vi "main.vi"() -> ()   [LabVIEW 2015]
panel:
  in  "stop":bool
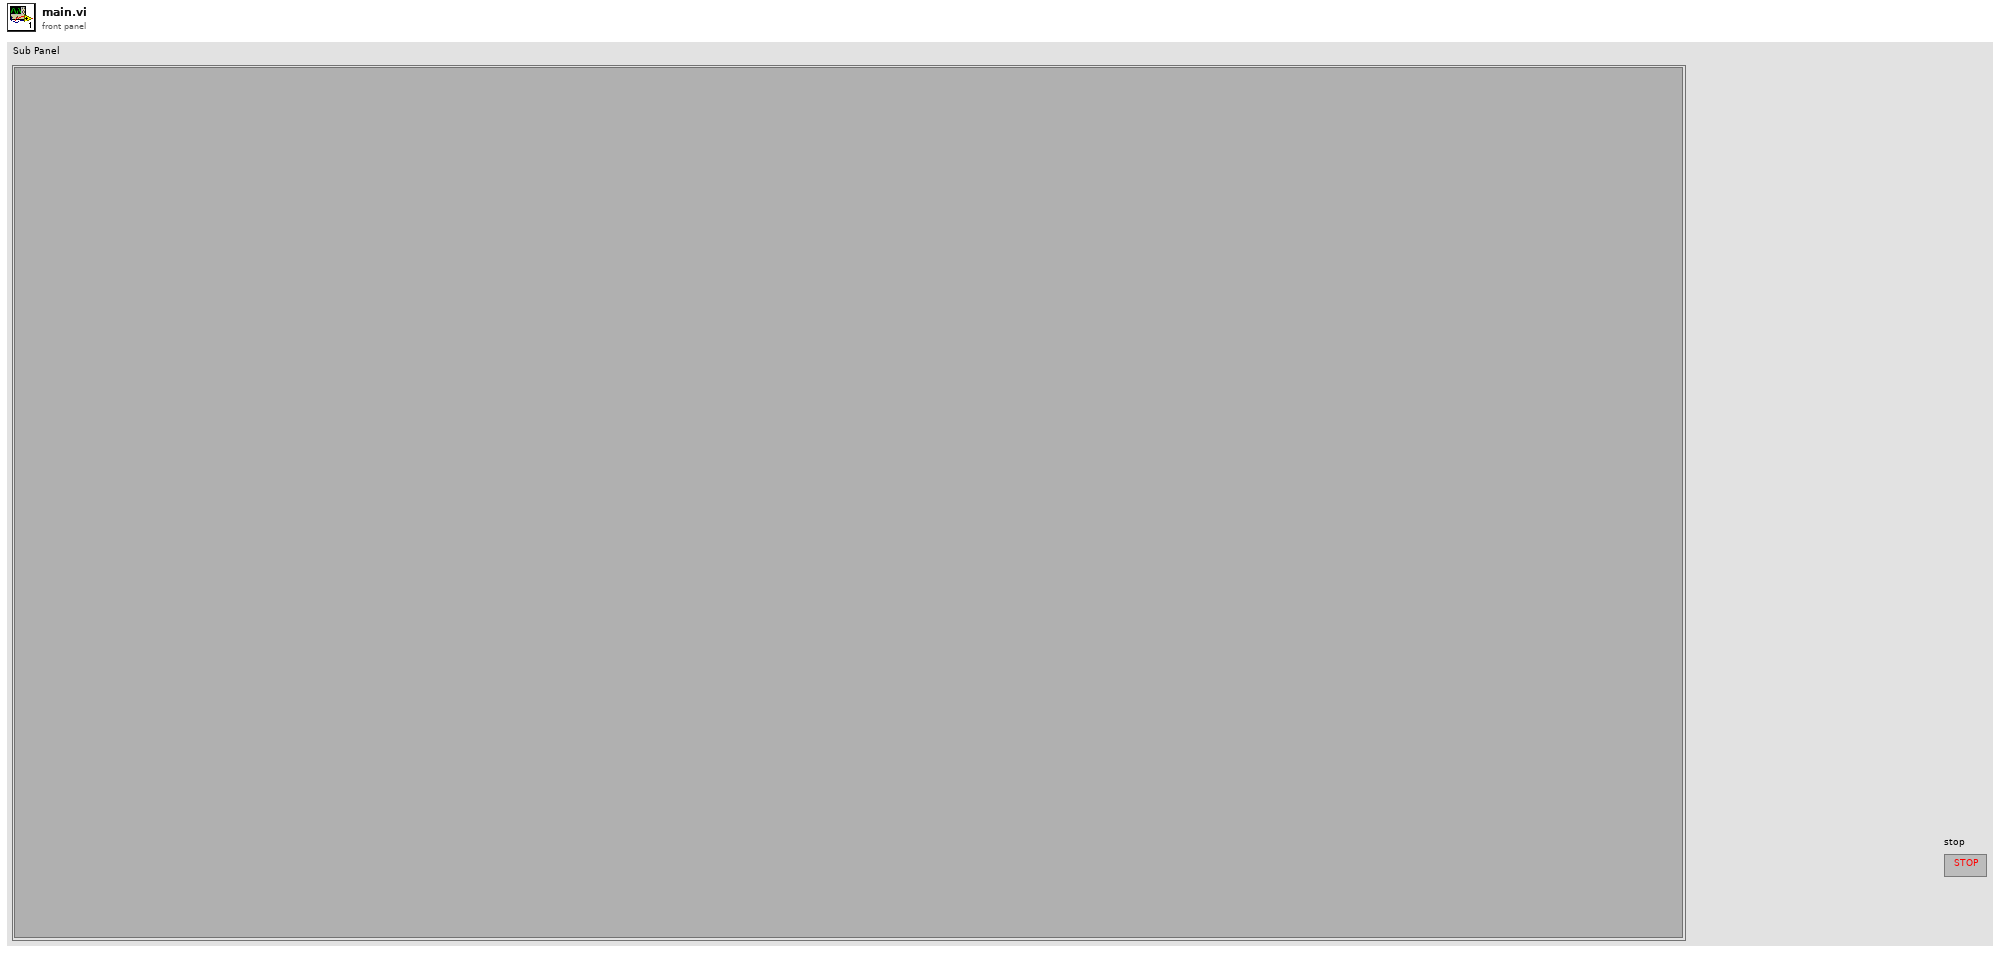
[diagram p1: front panel]
types:
  T1 = enum32{"Bad", "Idle", "Run top level", "Running"}
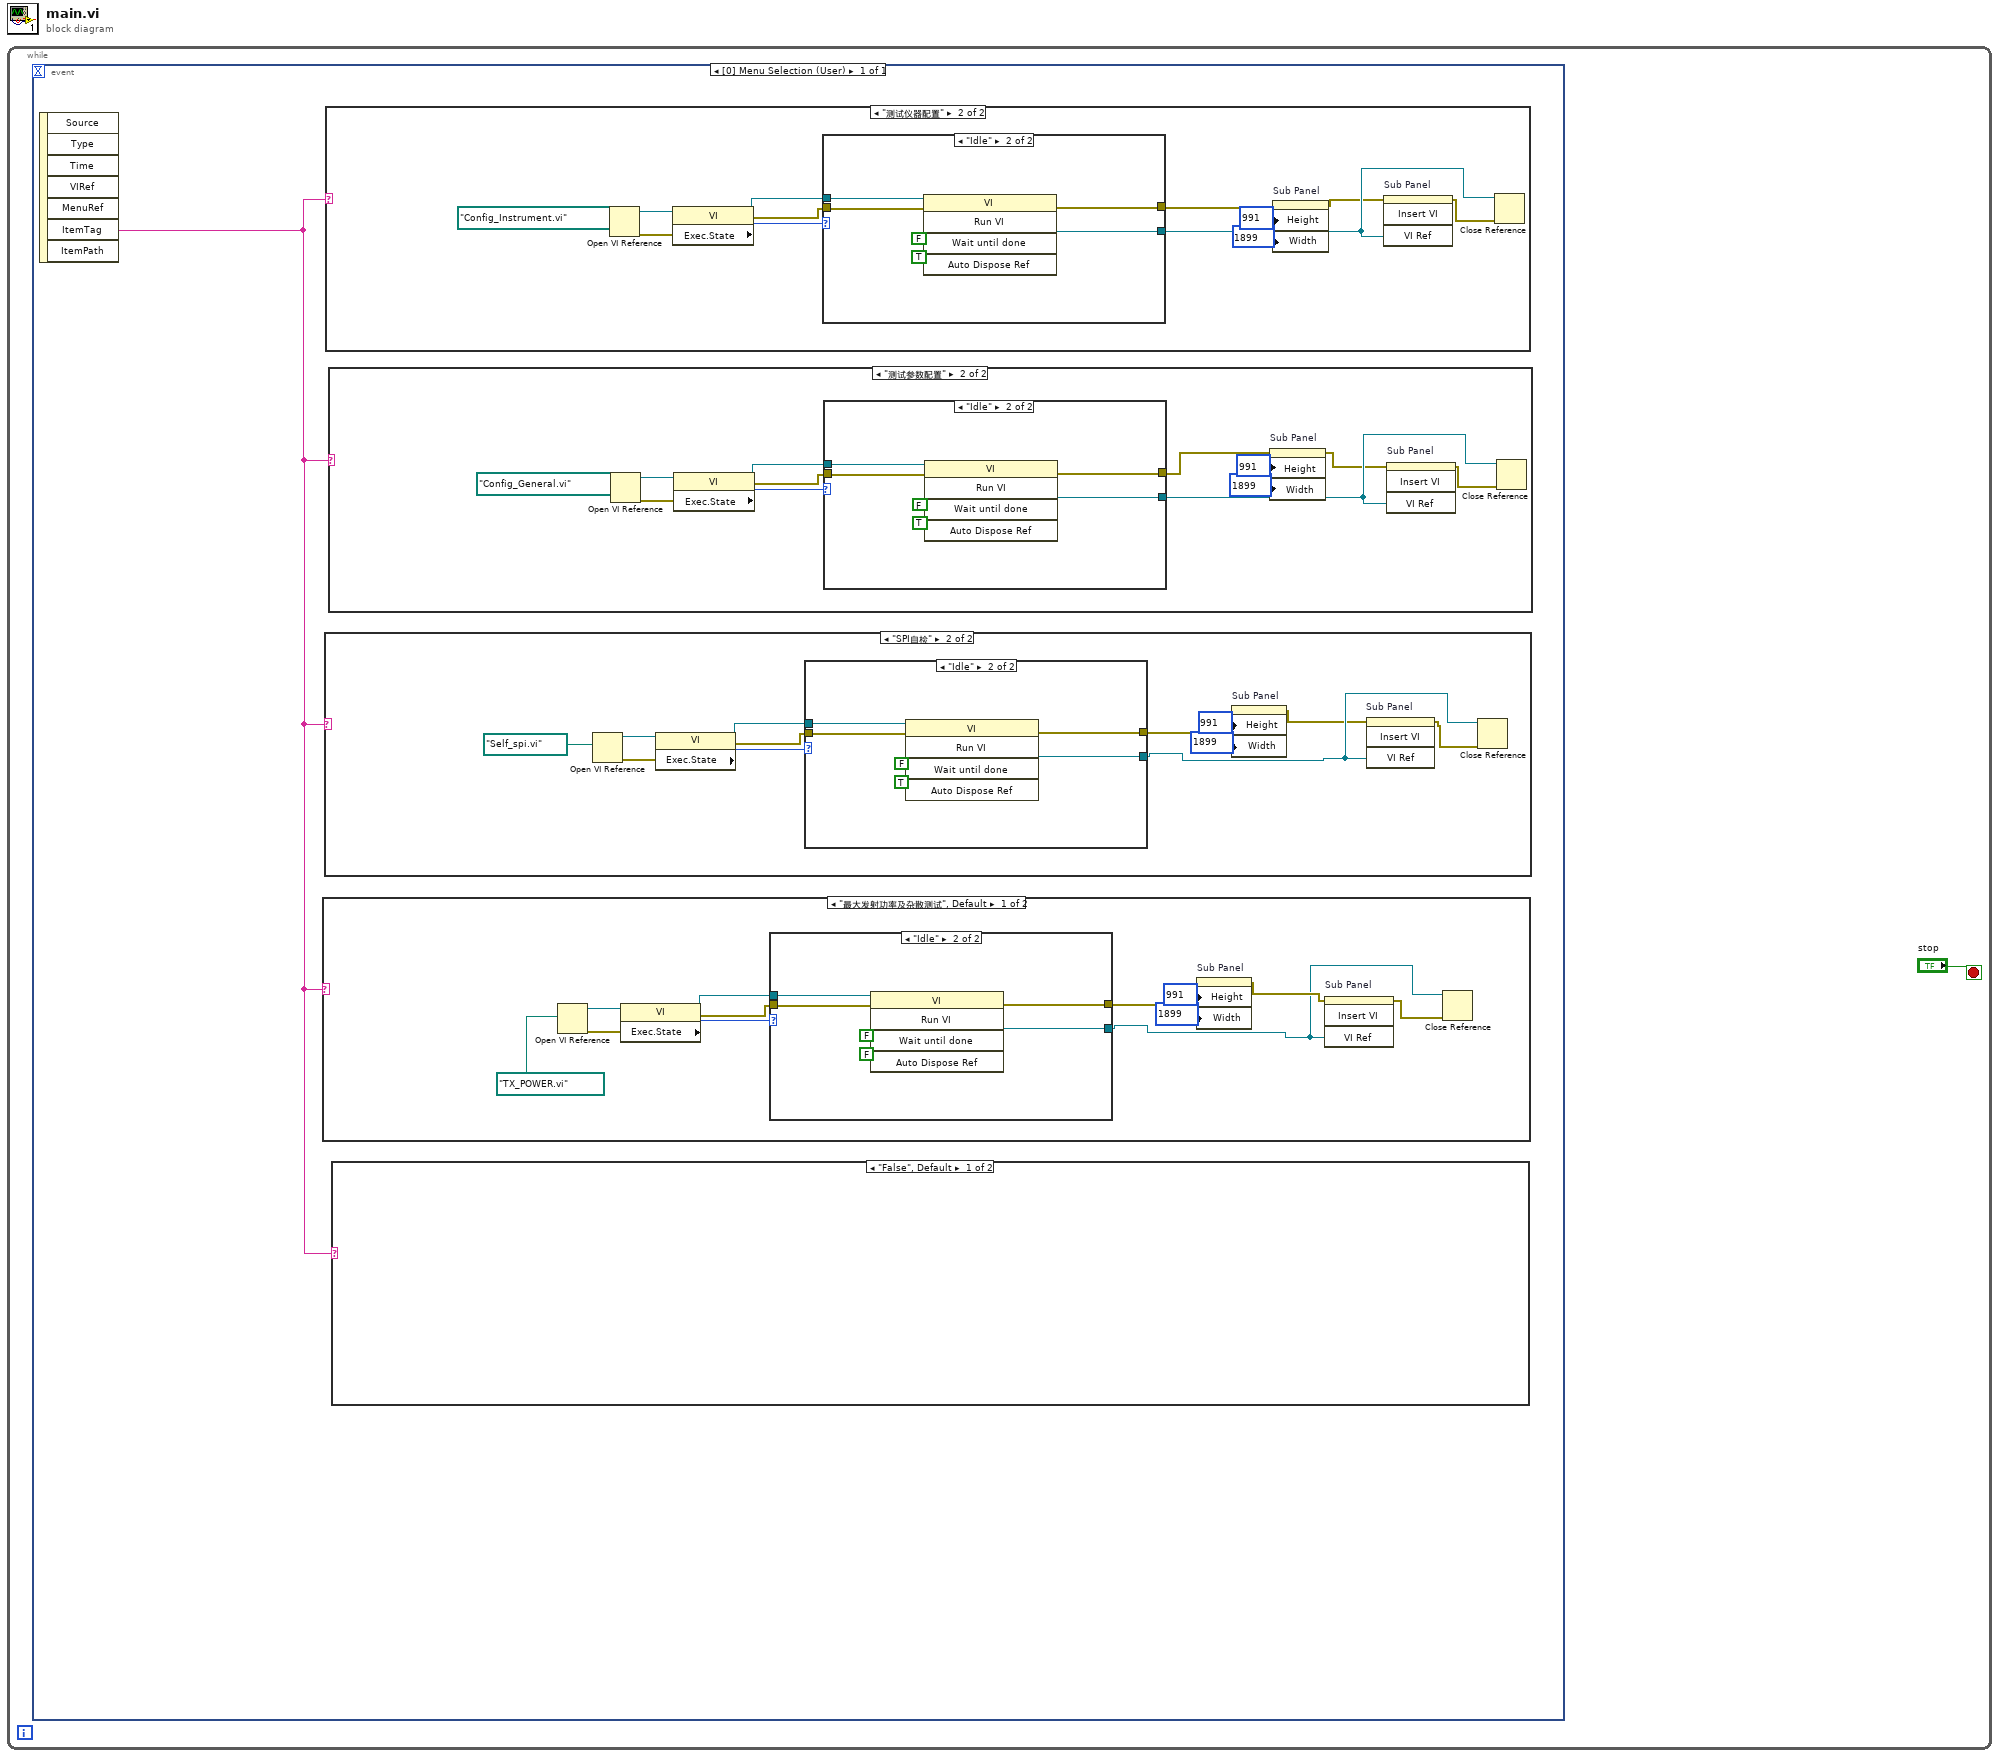
[diagram p0: block diagram]
diagram:
  n1 = while {
    stop <- "stop" stop-if-true
    n2 = event shown="[0] Menu Selection (User)" {
      selector: _ -> [_]
      dyn-events: _ -> [_]
      timeout: _ -> [_]
      event Menu Selection (User) {
        n3 = event-data() -> ("ItemTag"=w2:string)  [unwired: 1 in, 6 out]
        n4 = case shown="\"最大发射功率及杂散测试\", Default" w2 {
          frame "最大发射功率及杂散测试", Default {
            n5 = Open VI Reference(vi path=path "TX_POWER.vi") -> (vi reference=w6:refnum<vi>, error out=w8:errorcluster)  [unwired: 5 in]
            n6 = property class="VI"(reference=w6, error in=w8) -> (reference out=w9:refnum<vi>, error out=w10:errorcluster, "Exec.State"=w7:T1)
            n7 = case shown="\"Idle\"" w7 {
              tunnel: w9 -> [_ w20]
              tunnel: w10 -> [_ w19]
              tunnel: [_ w18] -> w12
              tunnel: [_ w17] -> w3
              frame "Bad", Default {
              }
              frame "Idle" {
                n8 = invoke class="VI" method="Run VI"(reference=w20, error in=w19, "Wait until done"=FALSE ("Wait Until Done"), "Auto Dispose Ref"=FALSE ("Auto Dispose Reference")) -> (reference out=w17:refnum<vi>, error out=w18:errorcluster)  [unwired: 1 in, 3 out]
              }
            }
            n9 = property on="Sub Panel" class="SubPnl"(error in=w12, "Height"=u32 991 ("Container Bounds:Height"), "Width"=u32 1899 ("Container Bounds:Width")) -> (error out=w5:errorcluster)  [unwired: 1 in, 1 out]
            n10 = invoke on="Sub Panel" class="SubPnl" method="Insert VI"(error in=w5, "VI Ref"=w3) -> (error out=w4:errorcluster)  [unwired: 2 in, 3 out]
            n11 = Close Reference(reference=w3, error in (no error)=w4) -> ()  [unwired: 1 out]
          }
          frame "2" {
          }
        }
        n12 = case shown="\"SPI自检\"" w2 {
          frame "False", Default {
          }
          frame "SPI自检" {
            n13 = Open VI Reference(vi path=path "Self_spi.vi") -> (vi reference=w32:refnum<vi>, error out=w30:errorcluster)  [unwired: 5 in]
            n14 = property class="VI"(reference=w32, error in=w30) -> (reference out=w29:refnum<vi>, error out=w28:errorcluster, "Exec.State"=w31:T1)
            n15 = case shown="\"Idle\"" w31 {
              tunnel: w29 -> [_ w38]
              tunnel: w28 -> [_ w37]
              tunnel: [_ w36] -> w24
              tunnel: [_ w35] -> w25
              frame "Bad", Default {
              }
              frame "Idle" {
                n16 = invoke class="VI" method="Run VI"(reference=w38, error in=w37, "Wait until done"=FALSE ("Wait Until Done"), "Auto Dispose Ref"=TRUE ("Auto Dispose Reference")) -> (reference out=w35:refnum<vi>, error out=w36:errorcluster)  [unwired: 1 in, 3 out]
              }
            }
            n17 = property on="Sub Panel" class="SubPnl"(error in=w24, "Height"=u32 991 ("Container Bounds:Height"), "Width"=u32 1899 ("Container Bounds:Width")) -> (error out=w23:errorcluster)  [unwired: 1 in, 1 out]
            n18 = invoke on="Sub Panel" class="SubPnl" method="Insert VI"(error in=w23, "VI Ref"=w25) -> (error out=w26:errorcluster)  [unwired: 2 in, 3 out]
            n19 = Close Reference(reference=w25, error in (no error)=w26) -> ()  [unwired: 1 out]
          }
        }
        n20 = case shown="\"测试仪器配置\"" w2 {
          frame "False", Default {
          }
          frame "测试仪器配置" {
            n21 = Open VI Reference(vi path=path "Config_Instrument.vi") -> (vi reference=w43:refnum<vi>, error out=w45:errorcluster)  [unwired: 5 in]
            n22 = property class="VI"(reference=w43, error in=w45) -> (reference out=w46:refnum<vi>, error out=w47:errorcluster, "Exec.State"=w44:T1)
            n23 = case shown="\"Idle\"" w44 {
              tunnel: w46 -> [_ w56]
              tunnel: w47 -> [_ w55]
              tunnel: [_ w54] -> w42
              tunnel: [_ w53] -> w48
              frame "Bad", Default {
              }
              frame "Idle" {
                n24 = invoke class="VI" method="Run VI"(reference=w56, error in=w55, "Wait until done"=FALSE ("Wait Until Done"), "Auto Dispose Ref"=TRUE ("Auto Dispose Reference")) -> (reference out=w53:refnum<vi>, error out=w54:errorcluster)  [unwired: 1 in, 3 out]
              }
            }
            n25 = property on="Sub Panel" class="SubPnl"(error in=w42, "Height"=u32 991 ("Container Bounds:Height"), "Width"=u32 1899 ("Container Bounds:Width")) -> (error out=w41:errorcluster)  [unwired: 1 in, 1 out]
            n26 = invoke on="Sub Panel" class="SubPnl" method="Insert VI"(error in=w41, "VI Ref"=w48) -> (error out=w49:errorcluster)  [unwired: 2 in, 3 out]
            n27 = Close Reference(reference=w48, error in (no error)=w49) -> ()  [unwired: 1 out]
          }
        }
        n28 = case shown="\"测试参数配置\"" w2 {
          frame "False", Default {
          }
          frame "测试参数配置" {
            n29 = Open VI Reference(vi path=path "Config_General.vi") -> (vi reference=w66:refnum<vi>, error out=w64:errorcluster)  [unwired: 5 in]
            n30 = property class="VI"(reference=w66, error in=w64) -> (reference out=w63:refnum<vi>, error out=w62:errorcluster, "Exec.State"=w65:T1)
            n31 = case shown="\"Idle\"" w65 {
              tunnel: w63 -> [_ w74]
              tunnel: w62 -> [_ w73]
              tunnel: [_ w72] -> w60
              tunnel: [_ w71] -> w68
              frame "Bad", Default {
              }
              frame "Idle" {
                n32 = invoke class="VI" method="Run VI"(reference=w74, error in=w73, "Wait until done"=FALSE ("Wait Until Done"), "Auto Dispose Ref"=TRUE ("Auto Dispose Reference")) -> (reference out=w71:refnum<vi>, error out=w72:errorcluster)  [unwired: 1 in, 3 out]
              }
            }
            n33 = property on="Sub Panel" class="SubPnl"(error in=w60, "Height"=u32 991 ("Container Bounds:Height"), "Width"=u32 1899 ("Container Bounds:Width")) -> (error out=w59:errorcluster)  [unwired: 1 in, 1 out]
            n34 = invoke on="Sub Panel" class="SubPnl" method="Insert VI"(error in=w59, "VI Ref"=w68) -> (error out=w67:errorcluster)  [unwired: 2 in, 3 out]
            n35 = Close Reference(reference=w68, error in (no error)=w67) -> ()  [unwired: 1 out]
          }
        }
        n36 = case shown="\"False\", Default" w2 {
          frame "False", Default {
          }
          frame "3" {
          }
        }
      }
    }
  }
